vi "C4LV_openAllInterfaces.vi"(0 "c4hdl in":refnum<k24>, 11 "error in (no error)":errorcluster) -> (4 "c4hdl out":refnum<k24>, 6 "c4if Arr out":refnum<k24>[](array[refnum]), 15 "error out":errorcluster)   [LabVIEW 2015, in "libC4HdlLV.lvlib"]
uses:
  libC4HdlLV.lvlib
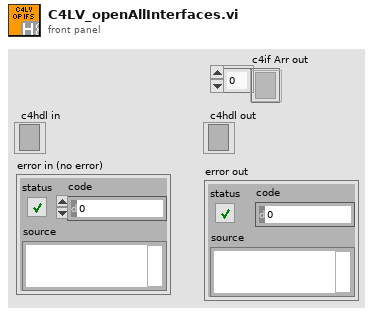
[diagram p1: front panel]
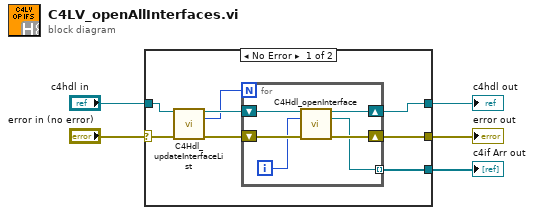
[diagram p0: block diagram]
diagram:
  n1 = case shown="No Error" "error in (no error)" {
    selector: "error in (no error)" -> [w10 w21]
    tunnel: "c4hdl in" -> [w8 w20]
    tunnel: [w12 w20] -> w2
    tunnel: [w13 w21] -> w5
    tunnel: [w11 _] -> w1
    frame No Error {
      n2 = call "C4Hdl_updateInterfaceList.vi"("c4hdl in"=w8, "error in (no error)"=w10) -> ("c4hdl out"=w7:refnum<k24>, "nofIf out"=w6:i64, "error out"=w9:errorcluster)  [unwired: 11 in]
      n3 = for {
        N: w6 -> [_]
        shift-right: [w18] -> w13
        shift-left: w9 -> [w19]
        shift-right: [w16] -> w12
        shift-left: w7 -> [w17]
        tunnel: [w14] -> w11 mode=indexing
        i -> [w15]
        n4 = call "C4Hdl_openInterface.vi"("c4hdl in"=w17, "ifNo in"=w15, "error in (no error)"=w19) -> ("c4hdl out"=w16:refnum<k24>, "c4if out"=w14:refnum<k24>, "error out"=w18:errorcluster)  [unwired: 10 in]
      }
    }
    frame Error {
    }
  }
  "error out" <- w5
  "c4hdl out" <- w2
  "c4if Arr out" <- w1
